vi "proc_handle_size.vi"(8 "error in":errorcluster) -> (0 "error out":errorcluster, 2 "size [B]":i32, 3 "new instance handle":u32[](array[numeric]))   [LabVIEW 2012]
doc: "Returns size of lv_process instance handler in bytes. Allocates memory for new instance handler if requiered."
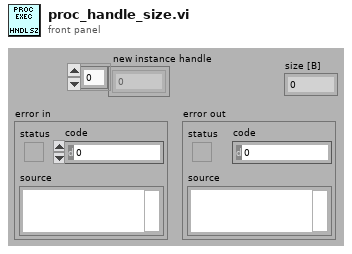
[diagram p1: front panel]
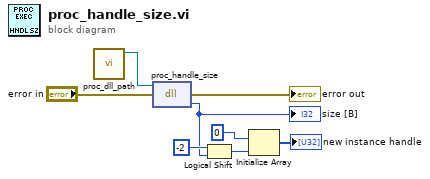
[diagram p0: block diagram]
diagram:
  n1 = call "proc_dll_path.vi"() -> ("path out"=w6:path)  [unwired: 10 in, 1 out]
  n2 = dll-call lib="lv_proc.dll" fn="proc_handle_size"(path in=w6, error in="error in") -> (error out=→"error out":errorcluster, "size [B]"=w1:i32)  [unwired: 1 in, 1 out]
  "size [B]" <- w1
  n3 = Logical Shift(y=-2 ("x"), x=w1) -> (x << y=w3:i32)
  n4 = Initialize Array(u32 0 ("element"), w3) -> (→"new instance handle":u32[])
